vi "Send Write Deadband.vi"(7 "消息优先级（标准）":T2=enum."Normal", 8 "error in (no error)":cluster{"状态":bool, "代码":i32, "源":string} caption="错误输入（无错误）", 10 "死区":T1, 11 "消息待入队列":refnum<class "Message Enqueuer.lvclass">) -> (0 "error out":cluster{"状态":bool, "代码":i32, "源":string} caption="错误输出")   [LabVIEW 2015, in "Level Controller.lvlib" / "Write Deadband Msg.lvclass"]
doc: "本VI将消息发送至操作者。输入为新的死区范围。关于“死区”的更多信息，见“水位控制器”类的说明信息。"
uses:
  Write Deadband Msg.lvclass
  <vilib>/ActorFramework/Message Enqueuer/Message Enqueuer.lvclass
  <vilib>/ActorFramework/Message Enqueuer/Message Priority.ctl
  Level Controller/Deadband.ctl
  Write Deadband Msg.lvclass/Write Deadband Msg.ctl
  <vilib>/ActorFramework/Message Enqueuer/Message Enqueuer.lvclass/Message Enqueuer.ctl
  <vilib>/ActorFramework/Message Priority Queue/Priority Enqueue.vi
  Level Controller/Level Controller.lvclass
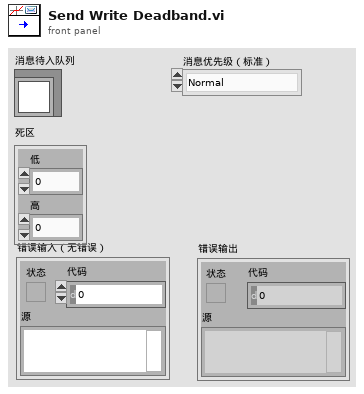
[diagram p1: front panel]
types:
  T1 = typedef "Level Controller.lvlib/Level Controller.lvclass/Deadband.ctl" = cluster{"低":dbl, "高":dbl}
  T2 = typedef "Actor Framework.lvlib/Message Enqueuer.lvclass/Message Priority.ctl" = enum16{"Low", "Normal", "High"}
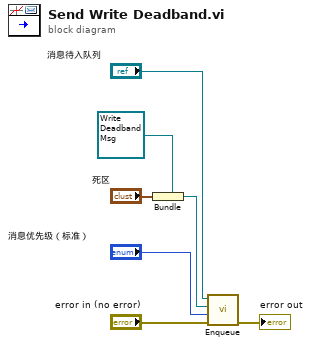
[diagram p0: block diagram]
diagram:
  n1 = Bundle(cluster=refnum<class "Write Deadband Msg.lvclass"> refnum ("Object"), "死区") -> (w3:refnum<class "Write Deadband Msg.lvclass">)
  n2 = call <vilib>:"Enqueue.vi"("error in (no error)"="error in (no error)", "Message Priority (Normal)"="消息优先级（标准）", "Message"=w3, "Message Enqueuer in"="消息待入队列") -> ("error out"=→"error out":errorcluster)  [unwired: 6 in, 1 out]
